vi "HCC Reformat Current Data to String Array.vi"(9 "Station IDs":string[](array[string]), 10 "Names":string[](array[string]), 11 "Sorted Data":dbl[](array[numeric])) -> (3 "Current Array":string[][](array[string]))   [LabVIEW 2018]
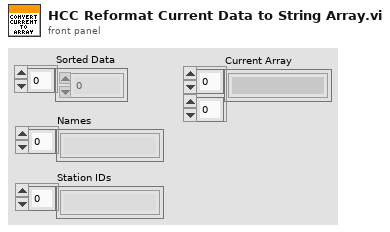
[diagram p1: front panel]
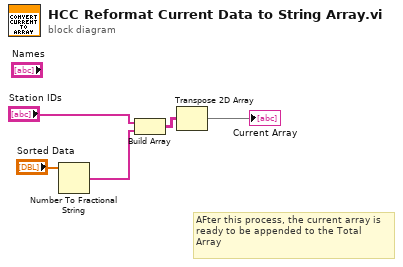
[diagram p0: block diagram]
diagram:
  # "AFter this process, the current array is\nready to be appended to the Total \nArray"
  n1 = Number To Fractional String(number="Sorted Data") -> (F-format string=w2:string[])  [unwired: 3 in]
  n2 = Build Array("Station IDs", w2) -> (w4:string[][])
  n3 = Transpose 2D Array(2D array=w4) -> (transposed array=→"Current Array":string[][])
